vi "Convert_ChannelProperty_to_JSON.vi"(8 "error in (no error)":errorcluster, 11 "channelProperties":T1 {"channel" min=1 max=8 step=1}) -> (0 "error out":errorcluster, 3 "getChannelResponse":T8)   [LabVIEW 2019, in "Inst.KH7008.lvlib" / "Inst.Krohn-Hite-7008.lvclass"]
uses:
  Inst.Krohn-Hite-7008.lvclass
  Typedefs/getAllChannelsDatabase--Cluster.ctl
  KH7008/typedefs/channelProperties--Cluster.ctl
  KH7008/typedefs/channel--numeric.ctl
  KH7008/typedefs/gain--enum.ctl
  KH7008/typedefs/Input--Enum.ctl
  KH7008/typedefs/shunt--enum.ctl
  KH7008/typedefs/couple--Enum.ctl
  KH7008/typedefs/Filter--Enum.ctl
  KH7008/KH7008.lvlib
panel:
  out "device_id":string
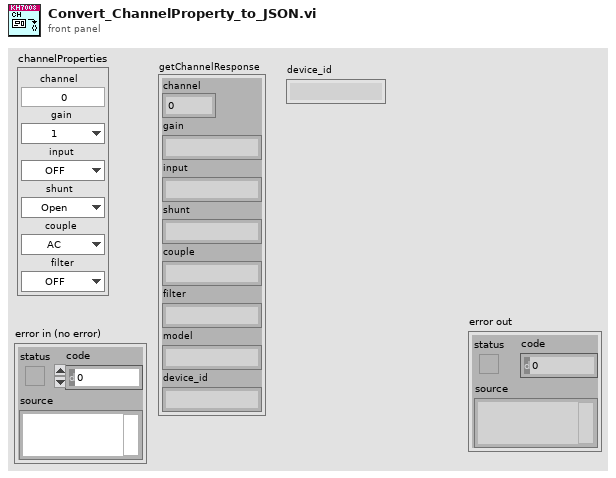
[diagram p1: front panel]
types:
  T1 = typedef "KH7008.lvlib/channelProperties--Cluster.ctl" = cluster{"channel":T2, "gain":T3, "input":T4, "shunt":T5, "couple":T6, "filter":T7}
  T2 = typedef "KH7008.lvlib/channel--numeric.ctl" = u16
  T3 = typedef "KH7008.lvlib/gain--enum.ctl" = enum16{"1", "10", "100", "1000"}
  T4 = typedef "KH7008.lvlib/input--enum.ctl" = enum16{"OFF", "SE+", "SE-", "DIFF"}
  T5 = typedef "KH7008.lvlib/shunt--enum.ctl" = enum16{"Open", "50", "500", "5k", "50k", "10M"}
  T6 = typedef "KH7008.lvlib/couple--enum.ctl" = enum16{"AC", "DC"}
  T7 = typedef "KH7008.lvlib/filter--enum.ctl" = enum16{"OFF", "ON"}
  T8 = typedef "Inst.KH7008.lvlib/Inst.Krohn-Hite-7008.lvclass/getAllChannelsDatabase--Cluster.ctl" = cluster{"channel":u32, "gain":string, "input":string, "shunt":string, "couple":string, "filter":string, "model":string, "device_id":string}
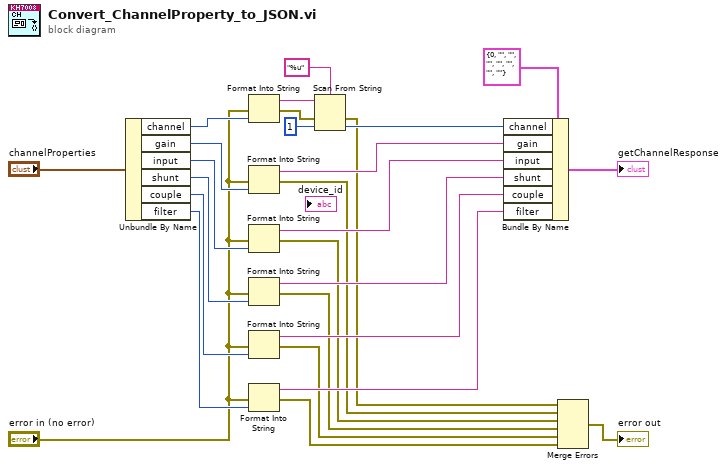
[diagram p0: block diagram]
diagram:
  n1 = Unbundle By Name("channelProperties") -> ("channel"=w24:T2, "gain"=w25:T3, "input"=w23:T4, "shunt"=w22:T5, "couple"=w21:T6, "filter"=w20:T7)
  n2 = Format Into String(error in="error in (no error)", w24) -> (resulting string=w16:string, error out=w8:errorcluster)  [unwired: 2 in]
  n3 = Format Into String(error in="error in (no error)", w25) -> (resulting string=w27:string, error out=w6:errorcluster)  [unwired: 2 in]
  n4 = Format Into String(error in="error in (no error)", w23) -> (resulting string=w13:string, error out=w5:errorcluster)  [unwired: 2 in]
  n5 = Format Into String(error in="error in (no error)", w22) -> (resulting string=w26:string, error out=w4:errorcluster)  [unwired: 2 in]
  n6 = Format Into String(error in="error in (no error)", w21) -> (resulting string=w15:string, error out=w3:errorcluster)  [unwired: 2 in]
  n7 = Format Into String(error in="error in (no error)", w20) -> (resulting string=w14:string, error out=w2:errorcluster)  [unwired: 2 in]
  n8 = Scan From String(format string="%u", input string=w16, error in=w8, default 1=u32 1 ("default value 1")) -> (error out=w7:errorcluster, output 1=w18:u32)  [unwired: 1 in, 2 out]
  n9 = Bundle By Name(cluster=T8 {"channel"=0, "gain"="", "input"="", "shunt"="", "couple"="", "filter"="", "model"="", "device_id"=""} ("getAllChannelsResponse"), "channel"=w18, "gain"=w27, "input"=w13, "shunt"=w26, "couple"=w15, "filter"=w14) -> (→"getChannelResponse":T8)
  n10 = Merge Errors(w7, w6, w5, w4, w3, w2) -> (→"error out":errorcluster)
